vi "DoHandshake.vi"(8 "error in (no error)":errorcluster, 9 "timeout ms (25000)":i32, 11 "TCP Network Connection in":refnum<k5>) -> (0 "error out":errorcluster, 2 "Headers Out":variant, 3 "TCP Network Connection out":refnum<k5>)   [LabVIEW 2013, in "WebSockets.lvlib"]
doc: "Performs the WebSockets HTTP handshaking on the new TCP connection. The client sends HTTP headers and the server must reply with a correctly formed HTTP response."
uses:
  WebSockets.lvlib
panel:
  out "HTTP Headers":string
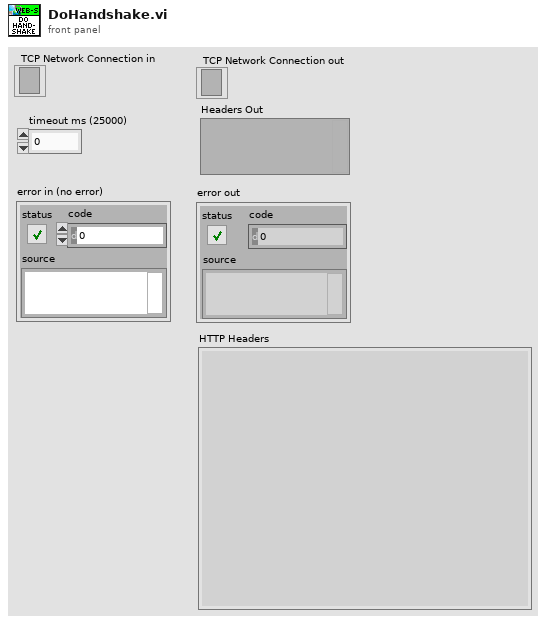
[diagram p1: front panel]
types:
  T1 = enum16{"Standard", "Buffered", "CRLF", "Immediate"}
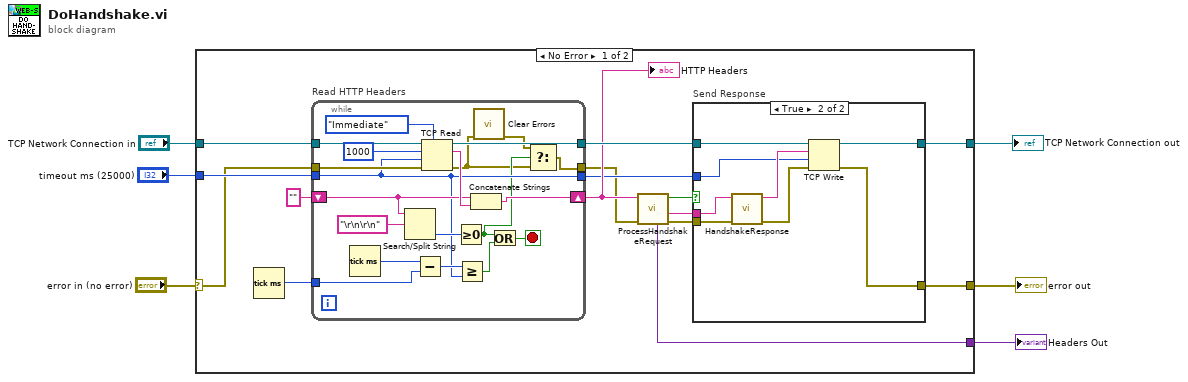
[diagram p0: block diagram]
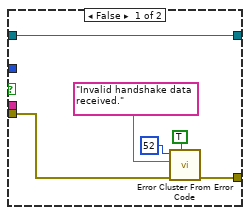
[diagram p2: hidden frame]
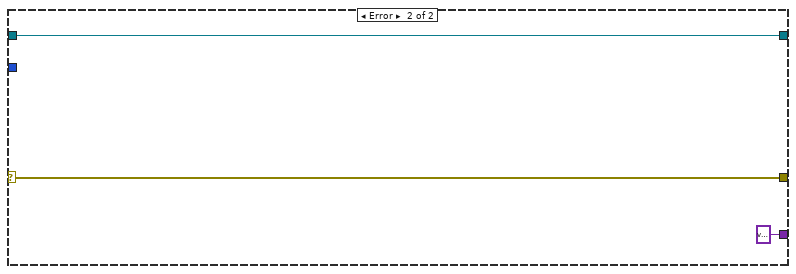
[diagram p3: hidden frame]
diagram:
  n1 = case shown="No Error" "error in (no error)" {
    selector: "error in (no error)" -> [w9 w58]
    tunnel: [w21 w57] -> w6
    tunnel: "TCP Network Connection in" -> [w15 w57]
    tunnel: [w13 w58] -> w3
    tunnel: "timeout ms (25000)" -> [w12 _]
    tunnel: [w7 variant ("Headers Out")] -> w1
    frame No Error {
      n2 = Tick Count (ms)() -> (millisecond timer value=w8:u32)
      n3 = while "Read HTTP Headers" {
        tunnel: w15 -> [w55]
        tunnel: [w54] -> w20
        shift-right: [w52] -> w17
        shift-left: "" -> [w49]
        tunnel: w12 -> [w42]
        tunnel: [w42] -> w11
        tunnel: [w36] -> w10
        tunnel: w9 -> [w50]
        tunnel: w8 -> [w43]
        stop <- w48 stop-if-true
        n4 = Tick Count (ms)() -> (millisecond timer value=w44:u32)
        n5 = Search/Split String(string=w49, search string/char (-)="\r\n\r\n") -> (offset of match=w47:i32)  [unwired: 1 in, 2 out]
        n6 = Subtract(x=w44, y=w43) -> (x-y=w46:u32)
        n7 = TCP Read(connection ID=w55, bytes to read=1000, error in (no error)=w50, 7:T1."Immediate" ("mode (standard)"), 9:w42) -> (connection ID out=w54:refnum<k5>, data out=w51:string, error out=w38:errorcluster)
        n8 = Greater Or Equal To 0?(x=w47) -> (x >= 0?=w39:bool)
        n9 = Greater Or Equal?(x=w46, y=w42) -> (x >= y?=w45:bool)
        n10 = Concatenate Strings(w49, w51) -> (w52:string)
        n11 = call <vilib>:"Clear Errors.vi"("error in (no error)"=w38) -> ("error out"=w37:errorcluster)  [unwired: 6 in]
        n12 = Or(x=w39, y=w45) -> (x .or. y?=w48:bool)
        n13 = Select(t=w37, s=w39, f=w38) -> (s? t:f=w36:errorcluster)
      }
      "HTTP Headers" <- w17
      n14 = call "ProcessHandshakeRequest.vi"("error in (no error)"=w10, "HTTP Headers"=w17) -> ("error out"=w14:errorcluster, "Sec-WebSocket-Key"=w19:string, "Is Websocket Request?"=w18:bool, "Headers Out"=w7:variant)  [unwired: 4 in, 2 out]
      n15 = case "Send Response" shown="True" w18 {
        tunnel: w19 -> [_ w35]
        tunnel: w20 -> [w27 w33]
        tunnel: [w27 w32] -> w21
        tunnel: w14 -> [w25 w30]
        tunnel: [w26 w29] -> w13
        tunnel: w11 -> [_ w28]
        frame False {
          n16 = call <vilib>:"Error Cluster From Error Code.vi"("show call chain? (False)"=TRUE, "error in (no error)"=w25, "error message (\"\")"="Invalid handshake data received." ("error message (\"\")"), "error code (0)"=52) -> ("error out"=w26:errorcluster)  [unwired: 5 in]
        }
        frame True {
          n17 = call "HandshakeResponse.vi"("error in (no error)"=w30, "Sec-WebSocket-Key"=w35) -> ("error out"=w31:errorcluster, "Response Headers"=w34:string)  [unwired: 8 in]
          n18 = TCP Write(connection ID=w33, data in=w34, error in (no error)=w31, 9:w28) -> (connection ID out=w32:refnum<k5>, error out=w29:errorcluster)  [unwired: 1 out]
        }
      }
    }
    frame Error {
    }
  }
  "TCP Network Connection out" <- w6
  "error out" <- w3
  "Headers Out" <- w1
